vi "Class Name.vi"(1 "LabVIEW Object":refnum<class>) -> (0 "Classname":string)   [LabVIEW 2009]
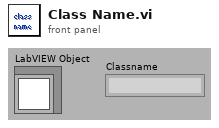
[diagram p1: front panel]
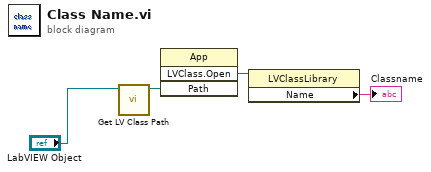
[diagram p0: block diagram]
diagram:
  n1 = call <vilib>:"Get LV Class Path.vi"("object"="LabVIEW Object") -> ("class path"=w2:path)  [unwired: 1 in, 9 out]
  n2 = invoke class="App" method="LVClass.Open"("Path"=w2) -> ("LVClass.Open"=w3:refnum<vi>)  [unwired: 3 in, 3 out]
  n3 = property class="LVClassLibrary"(reference=w3) -> ("Name"=→"Classname":string)  [unwired: 1 in, 2 out]
